vi "reflect.vi"(10 "N":dbl[](array[numeric]), 11 "I":dbl[](array[numeric])) -> (3 "Reflect":dbl[](array[numeric]))   [LabVIEW 2015]
uses:
  <vilib>/Analysis/baseanly.llb/Real Dot Product.vi
  <vilib>/Analysis/NI_AALBase.lvlib
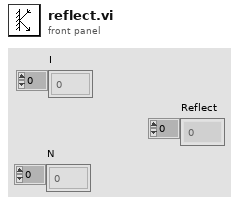
[diagram p1: front panel]
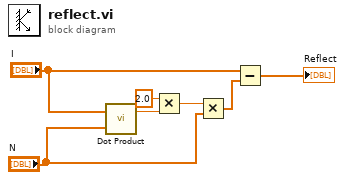
[diagram p0: block diagram]
diagram:
  n1 = call-poly <vilib>:"Dot Product.vi"("Y Vector"="N", "X Vector"="I") -> ("X * Y"=w7:dbl)  [unwired: 1 out]
  n2 = Multiply(x=2.0, y=w7) -> (x*y=w5:dbl)
  n3 = Multiply(x=w5, y="N") -> (x*y=w3:dbl[])
  n4 = Subtract(x="I", y=w3) -> (x-y=→"Reflect":dbl[])
